vi "CreateU3VHandle.vi"(7 "error in (no error)":errorcluster caption="错误输入（无错误）", 9 "U3VDevice":T1) -> (0 "error out":errorcluster caption="错误输出", 2 "handle":u64, 3 "function return":i32)   [LabVIEW 2011, in "MvCameraControl.lvlib"]
doc: "MV_LV_API int __stdcall CreateHandle(void ** handle, const MV_CC_DEVICE_INFO* pstDevInfo);"
uses:
  MvCameraControl.lvlib
  x86/MvCameraPatch.dll
types:
  T1 = cluster{"nMajorVer":u16, "nMinorVer":u16, "nMacAddrHigh":u32, "nMacAddrLow":u32, "nTLayerType":u32, "nReserved0":u32, "nReserved1":u32, "nReserved2":u32, "nReserved3":u32, "CrtlInEndPoint":u8, "CrtlOutEndPoint":u8, "StreamEndPoint":u8, "EventEndPoint":u8, "idVendor":u16, "idProduct":u16, "nDeviceNumber":u32, "nRes0":u32, "nRes1":u32, "chDeviceGUID":string, "chVendorName":string, "chModelName":string, "chFamilyName":string, "chDeviceVersion":string, "chManufacturerName":string, "chSerialNumber":string, "chUserDefinedName":string, "nbcdUSB":u32, "nRes2":u32, "nRes3":u32}
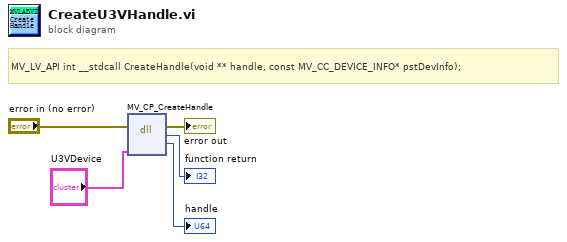
[diagram p0: block diagram]
diagram:
  # "MV_LV_API int __stdcall CreateHandle(void ** handle, const MV_CC_DEVICE_INFO* pstDevInfo);"
  n1 = dll-call lib="F:/SVN/SDK/Release/MVS/Samples/Labview/MvLVLib/x86/MvCameraPatch.dll" fn="MV_CP_CreateHandle"(error in="error in (no error)", "pstDevInfo"="U3VDevice") -> (error out=→"error out":errorcluster, "返回类型"=→"function return":i32, "handle"=→"handle":u64)  [unwired: 4 in, 1 out]
